vi "grid creator.vi"(0 "x-start":dbl, 3 "y-start":dbl) -> (15 "Output array":string[][](array[string]), 18 "Output string":string)   [LabVIEW 2018]
panel:
  in  "Create":bool
  in  "bidirectional":bool
  in  "x-first":bool
  in  "y-step":dbl=50.0
  in  "x-step":dbl=50.0
  in  "y-size":i32=5
  in  "x-size":i32=5
  # "SIM Control Grid Creator"
  # "unidirectional"
  # "y-first"
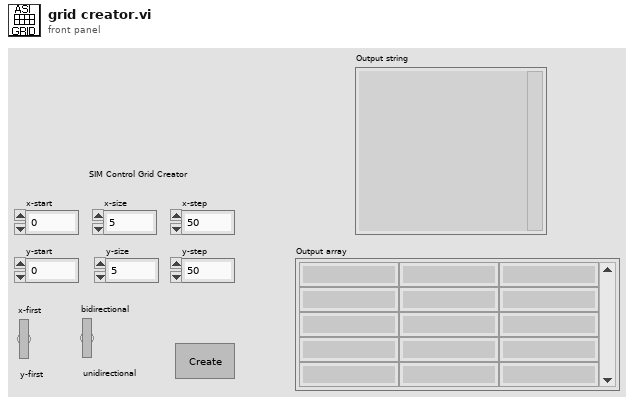
[diagram p1: front panel]
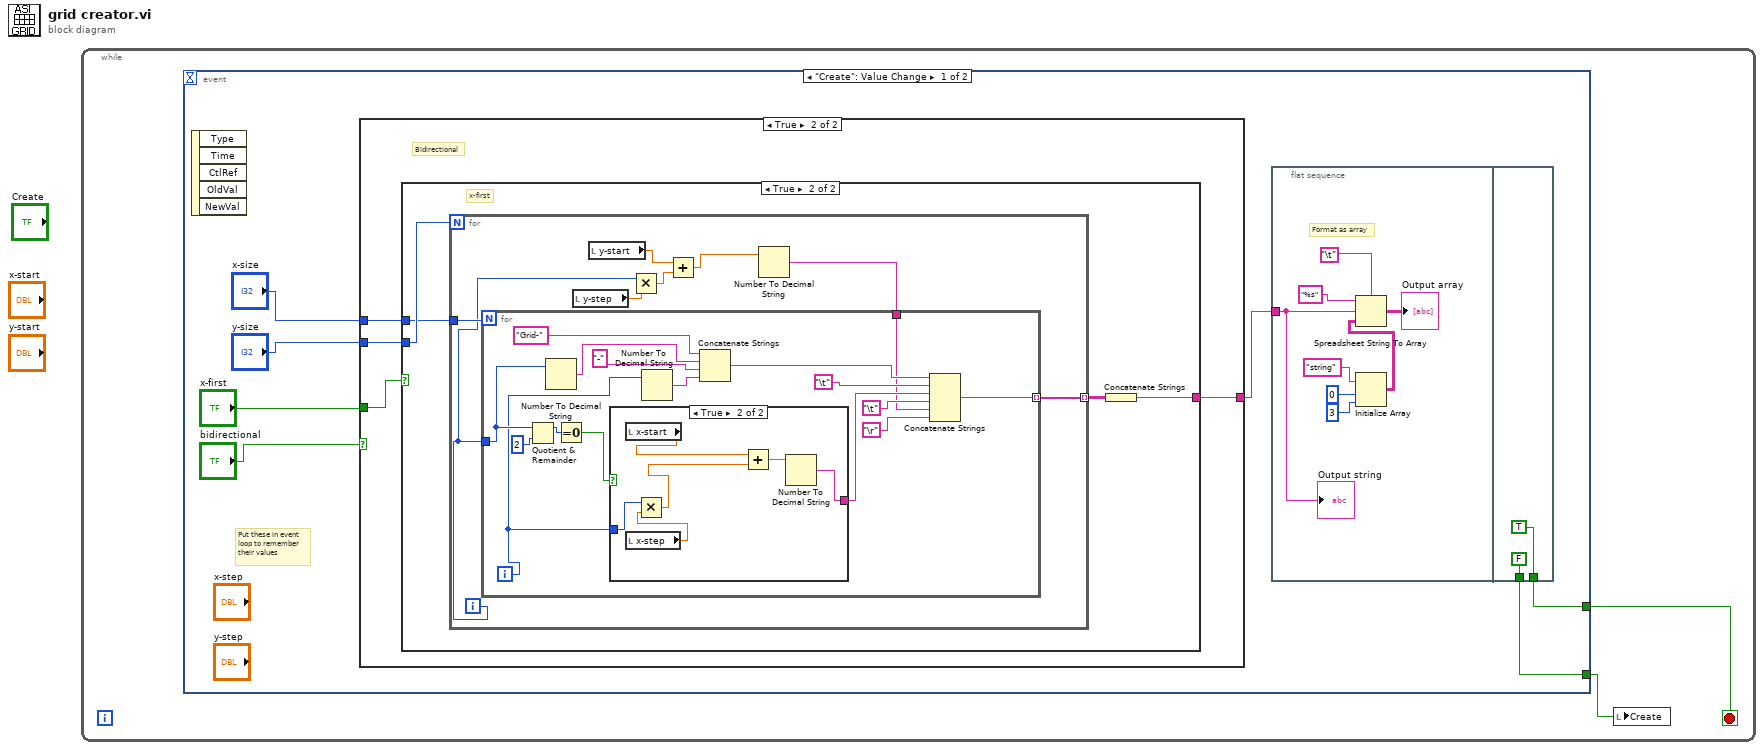
[diagram p0: block diagram]
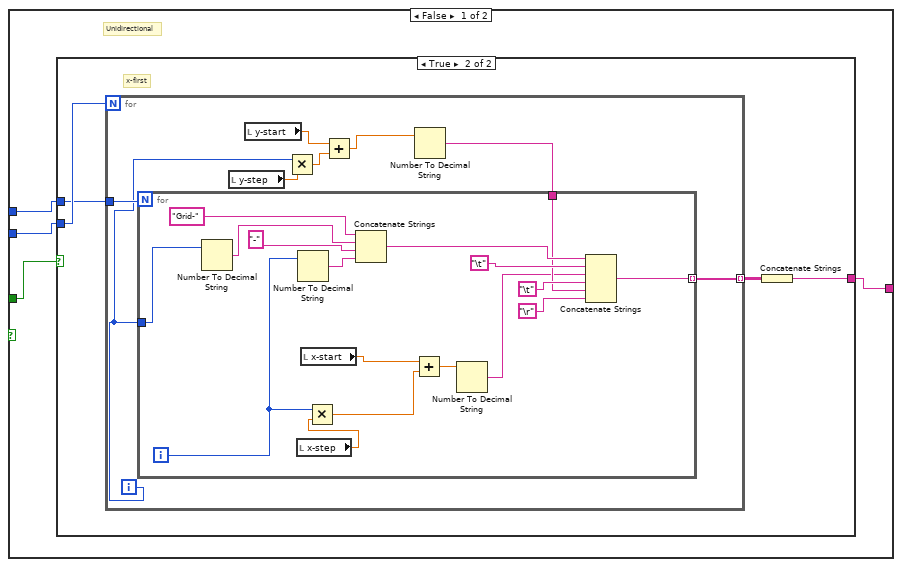
[diagram p2: hidden frame]
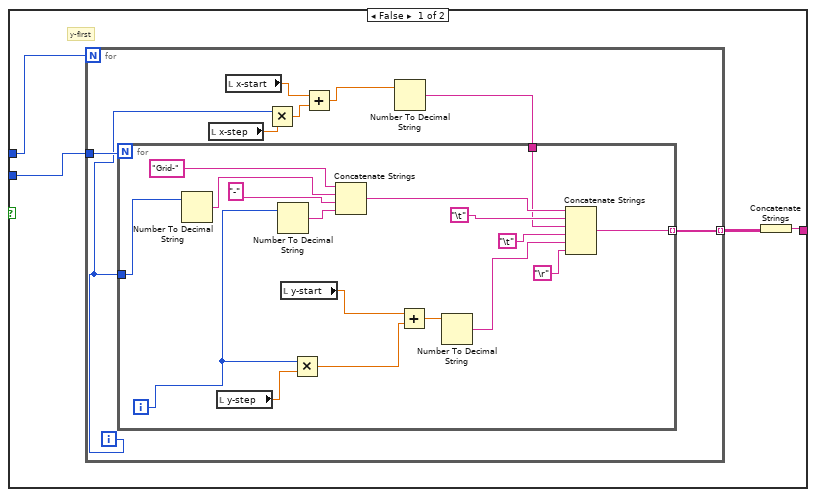
[diagram p3: hidden frame]
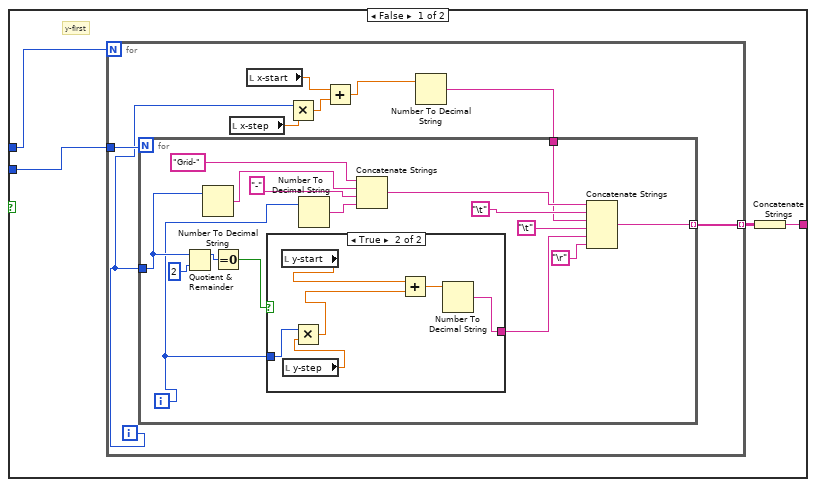
[diagram p4: hidden frame]
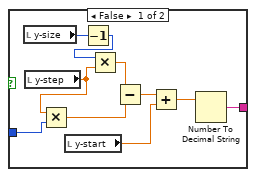
[diagram p5: hidden frame]
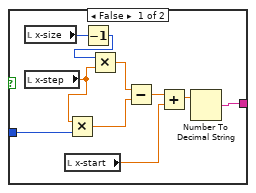
[diagram p6: hidden frame]
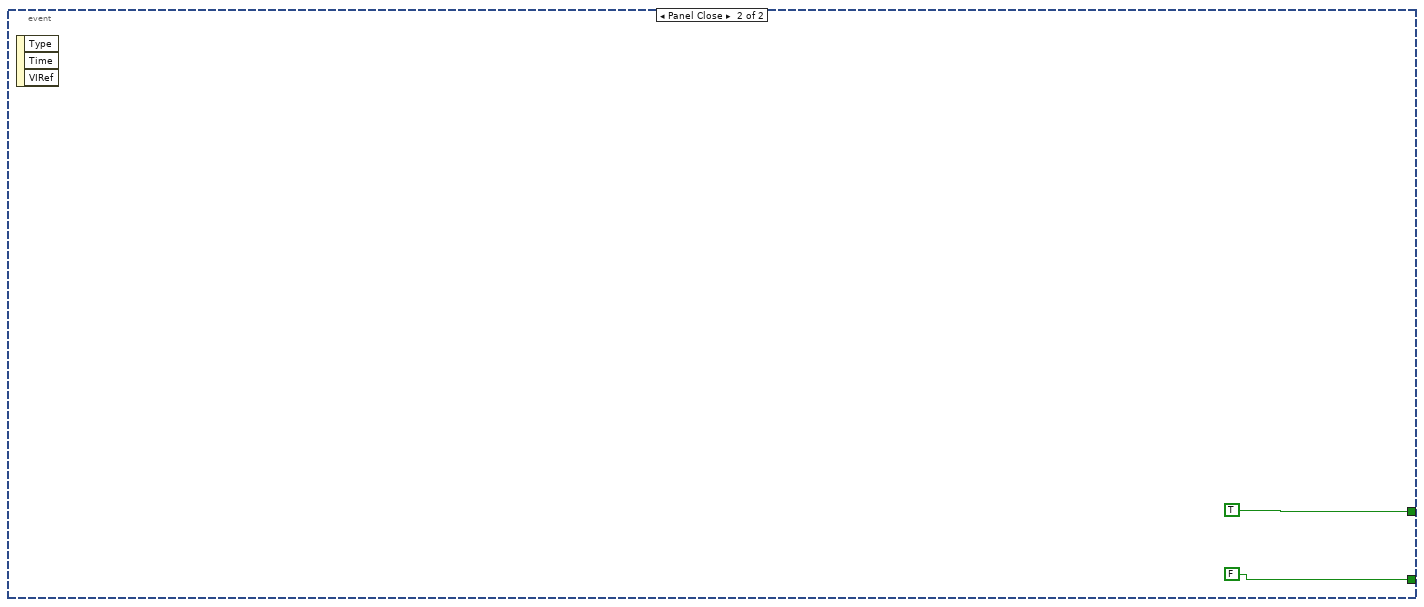
[diagram p7: hidden frame]
diagram:
  n1 = while {
    stop <- w2 stop-if-true
    n2 = event shown="[0] \"Create\": Value Change" {
      selector: _ -> [_ _]
      dyn-events: _ -> [_ _]
      timeout: _ -> [_ _]
      tunnel: [w8 TRUE] -> w2
      tunnel: [w7 FALSE] -> w1
      event "Create": Value Change {
        # "Put these in event\nloop to remember\ntheir values"
        n3 = event-data() -> ()  [unwired: 1 in, 5 out]
        n4 = case shown="True" "bidirectional" {
          tunnel: "x-first" -> [w20 w85]
          tunnel: "y-size" -> [w22 w84]
          tunnel: "x-size" -> [w21 w83]
          tunnel: [w23 w82] -> w9
          frame False {
            # "Unidirectional"
            n5 = case shown="True" w20 {
              tunnel: w22 -> [w26 w56]
              tunnel: w21 -> [w27 w55]
              tunnel: [w24 w53] -> w23
              frame False {
                # "y-first"
                n6 = for {
                  N: w27 -> [_]
                  tunnel: w26 -> [w35]
                  tunnel: [w28] -> w25 mode=indexing
                  i -> [w33]
                  n7 = local read "x-step"() -> (w34:dbl)
                  n8 = local read "x-start"() -> (w31:dbl)
                  n9 = Multiply(x=w33, y=w34) -> (x*y=w32:dbl)
                  n10 = Add(x=w31, y=w32) -> (x+y=w30:dbl)
                  n11 = Number To Decimal String(number=w30) -> (decimal integer string=w29:string)  [unwired: 1 in]
                  n12 = for {
                    N: w35 -> [_]
                    tunnel: w33 -> [w52]
                    tunnel: w29 -> [w37]
                    tunnel: [w43] -> w28 mode=indexing
                    i -> [w38]
                    n13 = Number To Decimal String(number=w52) -> (decimal integer string=w50:string)  [unwired: 1 in]
                    n14 = local read "y-step"() -> (w41:dbl)
                    n15 = Number To Decimal String(number=w38) -> (decimal integer string=w48:string)  [unwired: 1 in]
                    n16 = local read "y-start"() -> (w39:dbl)
                    n17 = Multiply(x=w38, y=w41) -> (x*y=w40:dbl)
                    n18 = Concatenate Strings("Grid-", w50, "-", w48) -> (w47:string)
                    n19 = Add(x=w39, y=w40) -> (x+y=w42:dbl)
                    n20 = Number To Decimal String(number=w42) -> (decimal integer string=w36:string)  [unwired: 1 in]
                    n21 = Concatenate Strings(w47, "\t", w37, "\t", w36, "\r") -> (w43:string)
                  }
                }
                n22 = Concatenate Strings(w25) -> (w24:string)
              }
              frame True {
                # "x-first"
                n23 = for {
                  N: w56 -> [_]
                  tunnel: w55 -> [w64]
                  tunnel: [w57] -> w54 mode=indexing
                  i -> [w62]
                  n24 = local read "y-step"() -> (w63:dbl)
                  n25 = local read "y-start"() -> (w60:dbl)
                  n26 = Multiply(x=w62, y=w63) -> (x*y=w61:dbl)
                  n27 = Add(x=w60, y=w61) -> (x+y=w59:dbl)
                  n28 = Number To Decimal String(number=w59) -> (decimal integer string=w58:string)  [unwired: 1 in]
                  n29 = for {
                    N: w64 -> [_]
                    tunnel: w62 -> [w81]
                    tunnel: w58 -> [w73]
                    tunnel: [w71] -> w57 mode=indexing
                    i -> [w67]
                    n30 = Number To Decimal String(number=w81) -> (decimal integer string=w79:string)  [unwired: 1 in]
                    n31 = local read "x-step"() -> (w66:dbl)
                    n32 = Number To Decimal String(number=w67) -> (decimal integer string=w77:string)  [unwired: 1 in]
                    n33 = local read "x-start"() -> (w65:dbl)
                    n34 = Multiply(x=w67, y=w66) -> (x*y=w69:dbl)
                    n35 = Concatenate Strings("Grid-", w79, "-", w77) -> (w76:string)
                    n36 = Add(x=w65, y=w69) -> (x+y=w70:dbl)
                    n37 = Number To Decimal String(number=w70) -> (decimal integer string=w68:string)  [unwired: 1 in]
                    n38 = Concatenate Strings(w76, "\t", w68, "\t", w73, "\r") -> (w71:string)
                  }
                }
                n39 = Concatenate Strings(w54) -> (w53:string)
              }
            }
          }
          frame True {
            # "Bidirectional"
            n40 = case shown="True" w85 {
              tunnel: w84 -> [w88 w133]
              tunnel: w83 -> [w89 w132]
              tunnel: [w86 w130] -> w82
              frame False {
                # "y-first"
                n41 = for {
                  N: w89 -> [_]
                  tunnel: w88 -> [w97]
                  tunnel: [w90] -> w87 mode=indexing
                  i -> [w95]
                  n42 = local read "x-step"() -> (w96:dbl)
                  n43 = local read "x-start"() -> (w93:dbl)
                  n44 = Multiply(x=w95, y=w96) -> (x*y=w94:dbl)
                  n45 = Add(x=w93, y=w94) -> (x+y=w92:dbl)
                  n46 = Number To Decimal String(number=w92) -> (decimal integer string=w91:string)  [unwired: 1 in]
                  n47 = for {
                    N: w97 -> [_]
                    tunnel: w95 -> [w113]
                    tunnel: w91 -> [w99]
                    tunnel: [w100] -> w90 mode=indexing
                    i -> [w109]
                    n48 = Quotient & Remainder(x=w113, y=2) -> (x-y*floor(x/y)=w111:i32)  [unwired: 1 out]
                    n49 = Number To Decimal String(number=w113) -> (decimal integer string=w107:string)  [unwired: 1 in]
                    n50 = Equal To 0?(x=w111) -> (x = 0?=w110:bool)
                    n51 = case shown="True" w110 {
                      tunnel: w109 -> [w121 w126]
                      tunnel: [w117 w124] -> w98
                      frame False {
                        n52 = local read "y-size"() -> (w123:i32)
                        n53 = local read "y-step"() -> (w120:dbl)
                        n54 = Multiply(x=w120, y=w121) -> (x*y=w118:dbl)
                        n55 = local read "y-start"() -> (w114:dbl)
                        n56 = Decrement(x=w123) -> (x-1=w122:i32)
                        n57 = Multiply(x=w122, y=w120) -> (x*y=w119:dbl)
                        n58 = Subtract(x=w119, y=w118) -> (x-y=w116:dbl)
                        n59 = Add(x=w116, y=w114) -> (x+y=w115:dbl)
                        n60 = Number To Decimal String(number=w115) -> (decimal integer string=w117:string)  [unwired: 1 in]
                      }
                      frame True {
                        n61 = local read "y-start"() -> (w129:dbl)
                        n62 = local read "y-step"() -> (w127:dbl)
                        n63 = Multiply(x=w126, y=w127) -> (x*y=w128:dbl)
                        n64 = Add(x=w129, y=w128) -> (x+y=w125:dbl)
                        n65 = Number To Decimal String(number=w125) -> (decimal integer string=w124:string)  [unwired: 1 in]
                      }
                    }
                    n66 = Number To Decimal String(number=w109) -> (decimal integer string=w105:string)  [unwired: 1 in]
                    n67 = Concatenate Strings("Grid-", w107, "-", w105) -> (w104:string)
                    n68 = Concatenate Strings(w104, "\t", w99, "\t", w98, "\r") -> (w100:string)
                  }
                }
                n69 = Concatenate Strings(w87) -> (w86:string)
              }
              frame True {
                # "x-first"
                n70 = for {
                  N: w133 -> [_]
                  tunnel: w132 -> [w141]
                  tunnel: [w134] -> w131 mode=indexing
                  i -> [w139]
                  n71 = local read "y-step"() -> (w140:dbl)
                  n72 = local read "y-start"() -> (w137:dbl)
                  n73 = Multiply(x=w139, y=w140) -> (x*y=w138:dbl)
                  n74 = Add(x=w137, y=w138) -> (x+y=w136:dbl)
                  n75 = Number To Decimal String(number=w136) -> (decimal integer string=w135:string)  [unwired: 1 in]
                  n76 = for {
                    N: w141 -> [_]
                    tunnel: w139 -> [w157]
                    tunnel: w135 -> [w144]
                    tunnel: [w142] -> w134 mode=indexing
                    i -> [w153]
                    n77 = Quotient & Remainder(x=w157, y=2) -> (x-y*floor(x/y)=w155:i32)  [unwired: 1 out]
                    n78 = Number To Decimal String(number=w157) -> (decimal integer string=w151:string)  [unwired: 1 in]
                    n79 = Equal To 0?(x=w155) -> (x = 0?=w154:bool)
                    n80 = case shown="True" w154 {
                      tunnel: w153 -> [w165 w170]
                      tunnel: [w161 w168] -> w146
                      frame False {
                        n81 = local read "x-size"() -> (w167:i32)
                        n82 = local read "x-step"() -> (w164:dbl)
                        n83 = local read "x-start"() -> (w158:dbl)
                        n84 = Multiply(x=w164, y=w165) -> (x*y=w162:dbl)
                        n85 = Decrement(x=w167) -> (x-1=w166:i32)
                        n86 = Multiply(x=w166, y=w164) -> (x*y=w163:dbl)
                        n87 = Subtract(x=w163, y=w162) -> (x-y=w159:dbl)
                        n88 = Add(x=w159, y=w158) -> (x+y=w160:dbl)
                        n89 = Number To Decimal String(number=w160) -> (decimal integer string=w161:string)  [unwired: 1 in]
                      }
                      frame True {
                        n90 = local read "x-start"() -> (w173:dbl)
                        n91 = local read "x-step"() -> (w171:dbl)
                        n92 = Multiply(x=w170, y=w171) -> (x*y=w172:dbl)
                        n93 = Add(x=w173, y=w172) -> (x+y=w169:dbl)
                        n94 = Number To Decimal String(number=w169) -> (decimal integer string=w168:string)  [unwired: 1 in]
                      }
                    }
                    n95 = Number To Decimal String(number=w153) -> (decimal integer string=w149:string)  [unwired: 1 in]
                    n96 = Concatenate Strings("Grid-", w151, "-", w149) -> (w148:string)
                    n97 = Concatenate Strings(w148, "\t", w146, "\t", w144, "\r") -> (w142:string)
                  }
                }
                n98 = Concatenate Strings(w131) -> (w130:string)
              }
            }
          }
        }
        n99 = flat-sequence {
          tunnel: w9 -> [w10]
          tunnel: [TRUE] -> w8
          tunnel: [FALSE] -> w7
          frame #0 {
            # "Format as array"
            n100 = Initialize Array("string" ("format string"), 0 ("dimension size"), 3 ("dimension size")) -> (w14:string[][])
            n101 = Spreadsheet String To Array(delimiter (Tab)="\t", format string="%s", spreadsheet string=w10, array type (2D Dbl)=w14) -> (array=→"Output array":string[][])
            "Output string" <- w10
          }
          frame #1 {
          }
        }
      }
      event Panel Close {
        n102 = event-data() -> ()  [unwired: 1 in, 3 out]
      }
    }
    n103 = local write "Create"(w1) -> ()
  }
